vi "test v70.vi"() -> ()   [LabVIEW 2020]
uses:
  <vilib>/Instr/_visa.llb/VISA Configure Serial Port (Instr).vi
panel:
  in  "OK Button":bool
  in  "stop":bool
  in  "V70 resource name":refnum<visa-resource-name>
  in  "V70 Write":string
  out "Response":string
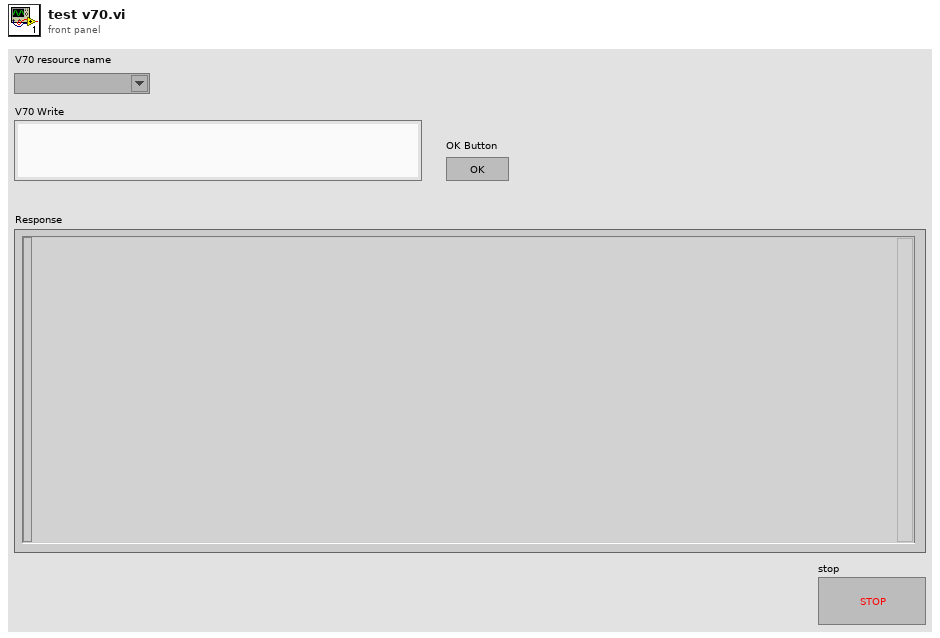
[diagram p1: front panel]
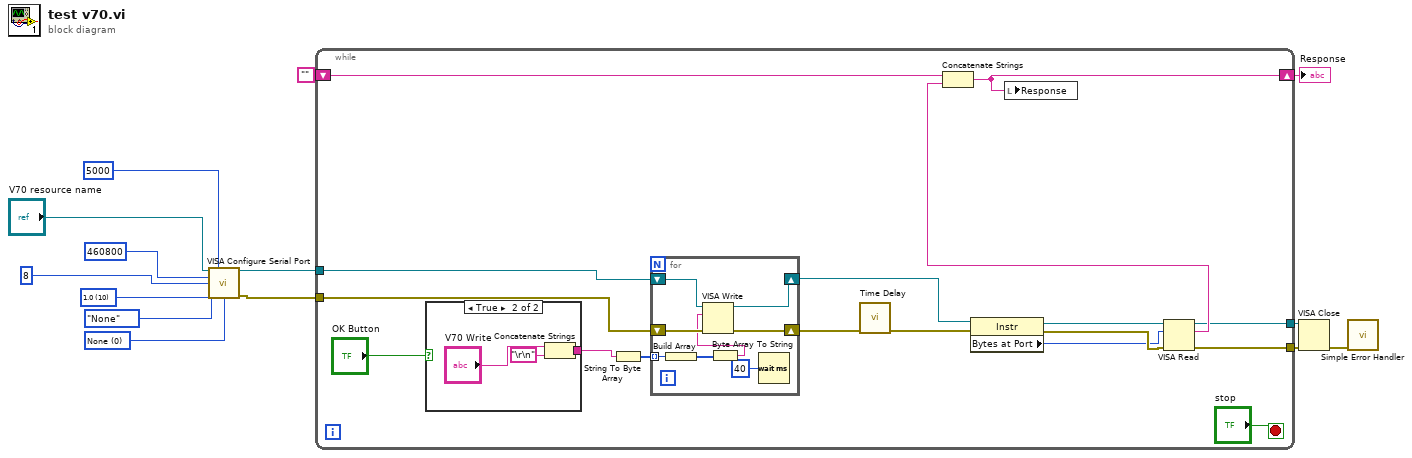
[diagram p0: block diagram]
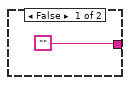
[diagram p2: hidden frame]
diagram:
  w11 = u16 0 items=["None", "XON/XOFF", "RTS/CTS", "XON/XOFF & RTS/CTS", "DTR/DSR", "XON/XOFF & DTR/DSR"] ("flow control (0:none)")
  w12 = u16 10 items=["1.0"=10, "1.5"=15, "2.0"=20] ("stop bits (10: 1 bit)")
  n1 = call-poly "VISA Configure Serial Port"("VISA resource name"="V70 resource name", "timeout (10sec)"=u32 5000, "baud rate (9600)"=u32 460800, "data bits (8)"=u16 8, "parity (0:none)"=enum16{"None", "Odd", "Even", "Mark", "Space"}."None", "stop bits (10: 1 bit)"=w12, "flow control (0:none)"=w11) -> ("VISA resource name out"=w2:refnum<visa-resource-name>, "error out"=w3:errorcluster)  [unwired: 2 in, 5 out]
  n2 = while {
    shift-right: [w29] -> w8
    shift-left: "" -> [w27]
    tunnel: [w25] -> w6
    tunnel: [w24] -> w5
    tunnel: w3 -> [w19]
    tunnel: w2 -> [w18]
    stop <- "stop" stop-if-true
    n3 = case shown="True" "OK Button" {
      tunnel: ["" w35] -> w20
      frame False {
      }
      frame True {
        n4 = Concatenate Strings("V70 Write", "\r\n") -> (w35:string)
      }
    }
    n5 = String To Byte Array(string=w20) -> (unsigned byte array=w21:u8[])
    n6 = for {
      shift-right: [w40] -> w17
      shift-left: w19 -> [w43]
      shift-right: [w41] -> w16
      shift-left: w18 -> [w42]
      tunnel: w21 -> [w39] mode=indexing
      n7 = Build Array(w39) -> (w38:u8[])
      n8 = Byte Array To String(unsigned byte array=w38) -> (string=w37:string)
      n9 = VISA Write(VISA resource name=w42, write buffer=w37, error in (no error)=w43) -> (VISA resource name out=w41:refnum<visa-resource-name>, error out=w40:errorcluster)  [unwired: 1 out]
      n10 = Wait (ms)(milliseconds to wait=u32 40) -> ()  [unwired: 1 out]
    }
    n11 = call "Time Delay"("error in (no error)"=w17) -> ("error out"=w26:errorcluster)  [unwired: 10 in]
    n12 = property class="Instr"(reference=w16, error in=w26) -> (reference out=w31:refnum<visa-resource-name>, error out=w30:errorcluster, "Bytes at Port"=w23:u32)
    n13 = VISA Read(VISA resource name=w31, byte count=w23, error in (no error)=w30) -> (VISA resource name out=w24:refnum<visa-resource-name>, read buffer=w28:string, error out=w25:errorcluster)  [unwired: 1 out]
    n14 = Concatenate Strings(w27, w28) -> (w29:string)
    n15 = local write "Response"(w29) -> ()
  }
  "Response" <- w8
  n16 = VISA Close(VISA resource name=w5, error in (no error)=w6) -> (error out=w4:errorcluster)
  n17 = call <vilib>:"Simple Error Handler.vi"("error in (no error)"=w4) -> ()  [unwired: 4 in, 5 out]
